vi "Save Test Executive.vi"(8 "error in (no error)":errorcluster, 10 "Path":path, 11 "Test Executive Builder in":refnum<class "Test Executive Builder.lvclass">) -> (0 "error out":errorcluster, 3 "Test Executive Builder out":refnum<class "Test Executive Builder.lvclass">)   [LabVIEW 2017, in "Test Executive Builder.lvclass"]
uses:
  Test Executive Builder.lvclass
  Source/Test Executive Builder Model/Test Executive Builder Model/Test Executive Builder Model.lvclass
  <vilib>/gpm_packages/@cs/mva-core/Source/IModel/IModel/IModel.lvclass
  C:/Users/jonmc/Documents/Git/Test Executive Builder/gpm_packages/@cs/mva-core/Source/IModel/IModel/IModel.lvclass
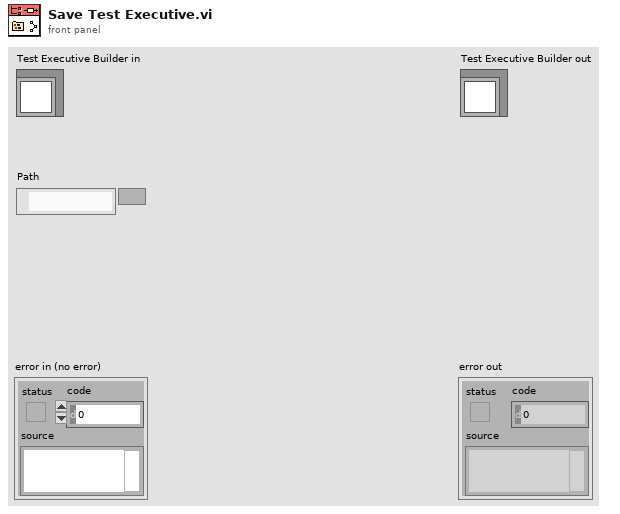
[diagram p1: front panel]
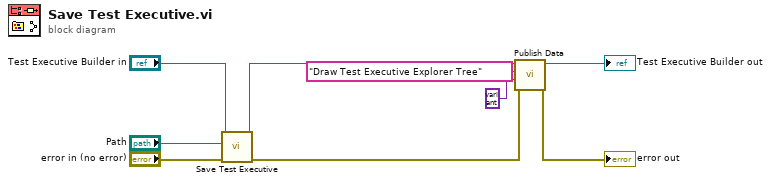
[diagram p0: block diagram]
diagram:
  n1 = call-parent "Save Test Executive.vi"("error in (no error)"="error in (no error)", "Path"="Path", "Test Executive Builder Model in"="Test Executive Builder in") -> ("error out"=w2:errorcluster, "Test Executive Builder Model out"=w4:refnum<class "Test Executive Builder.lvclass">)  [unwired: 7 in]
  n2 = call <vilib>:"Publish Data.vi"("error in (no error)"=w2, "Data to Publish"=variant ("Data Type"), "Datum Name"="Draw Test Executive Explorer Tree", "IModel in"=w4) -> ("error out"=→"error out":errorcluster, "IModel out"=→"Test Executive Builder out":refnum<class "Test Executive Builder.lvclass">)  [unwired: 6 in]
